vi "buildArray.vi"() -> ()   [LabVIEW 2021]
panel:
  out "appended array":dbl[][](array[numeric])
  in  "Array 3":dbl[](array[numeric])
  in  "Array 2":dbl[](array[numeric])
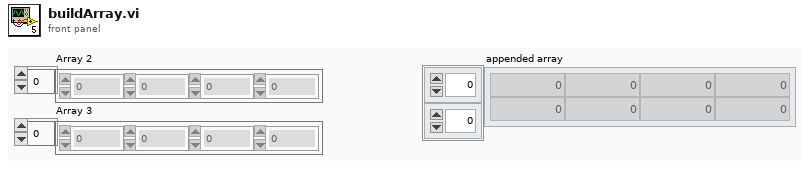
[diagram p1: front panel]
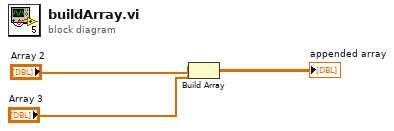
[diagram p0: block diagram]
diagram:
  n1 = Build Array "Build Array"("Array 2", "Array 3") -> (→"appended array":dbl[][])
